vi "MISC Match First Header.vi"(0 "Call Chain":string[](array[string]), 5 "Headers":string[](array[string]), 7 "Fulll Names":string[](array[string]), 9 "Default Name":string) -> (4 "Full Name":string)   [LabVIEW 2011]
doc: "This routine performs a find and replace on each element pair in the search and replace arrays."
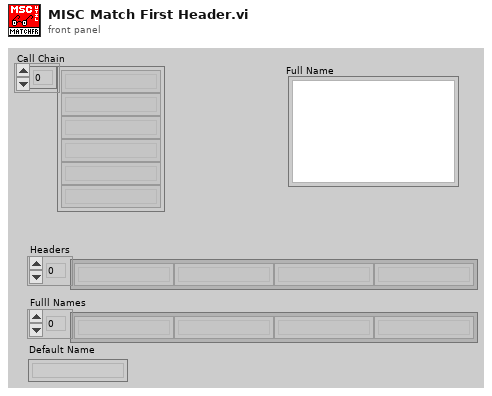
[diagram p1: front panel]
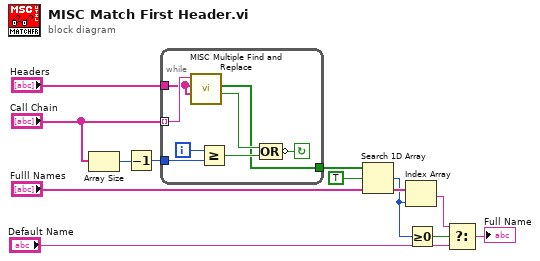
[diagram p0: block diagram]
diagram:
  n1 = Array Size(array="Call Chain") -> (size(s)=w12:i32)
  n2 = Decrement(x=w12) -> (x-1=w9:i32)
  n3 = while {
    tunnel: [w14] -> w11
    tunnel: w9 -> [w19]
    tunnel: "Call Chain" -> [w20] mode=indexing
    tunnel: "Headers" -> [w13]
    i -> [w18]
    stop <- w17 continue-if-true
    n4 = call "MISC Multiple Find and Replace.vi"("Replace Text Array"=w13, "Search Text Array"=w13, "Input String"=w20) -> ("Match"=w15:bool, "Matches"=w14:bool[])  [unwired: 7 out]
    n5 = Greater Or Equal?(x=w18, y=w19) -> (x >= y?=w16:bool)
    n6 = Compound Arithmetic op=OR(w15, w16) -> (invert w17:bool)
  }
  n7 = Search 1D Array(1D array=w11, element=TRUE) -> (index of element=w4:i32)  [unwired: 1 out]
  n8 = Index Array(array="Fulll Names", index=w4) -> (element=w2:string)
  n9 = Greater Or Equal To 0?(x=w4) -> (x >= 0?=w5:bool)
  n10 = Select(t=w2, s=w5, f="Default Name") -> (s? t:f=→"Full Name":string)
